vi "Task five.vi"() -> ()   [LabVIEW 2025]
uses:
  <vilib>/httpClient/POSTBuffer.vi
  <vilib>/httpClient/LabVIEWHTTPClient.lvlib
panel:
  in  "User Input":string
  in  "?":bool
  in  "Select correct word":string(combo)
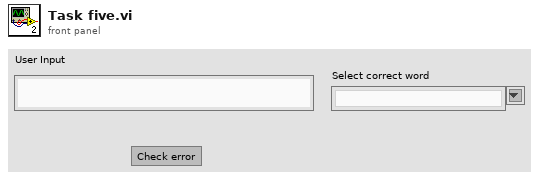
[diagram p1: front panel]
types:
  T1 = cluster{"matches":cluster{"offset":i32, "length":i32, "message":string, "replacements":cluster{"value":string}[]}[]}
  T2 = typedef "LabVIEWHTTPClient.lvlib/ClientHandle.ctl" = refnum<k1>
  T3 = cluster{"offset":i32, "length":i32, "message":string, "replacements":cluster{"value":string}[]}[]
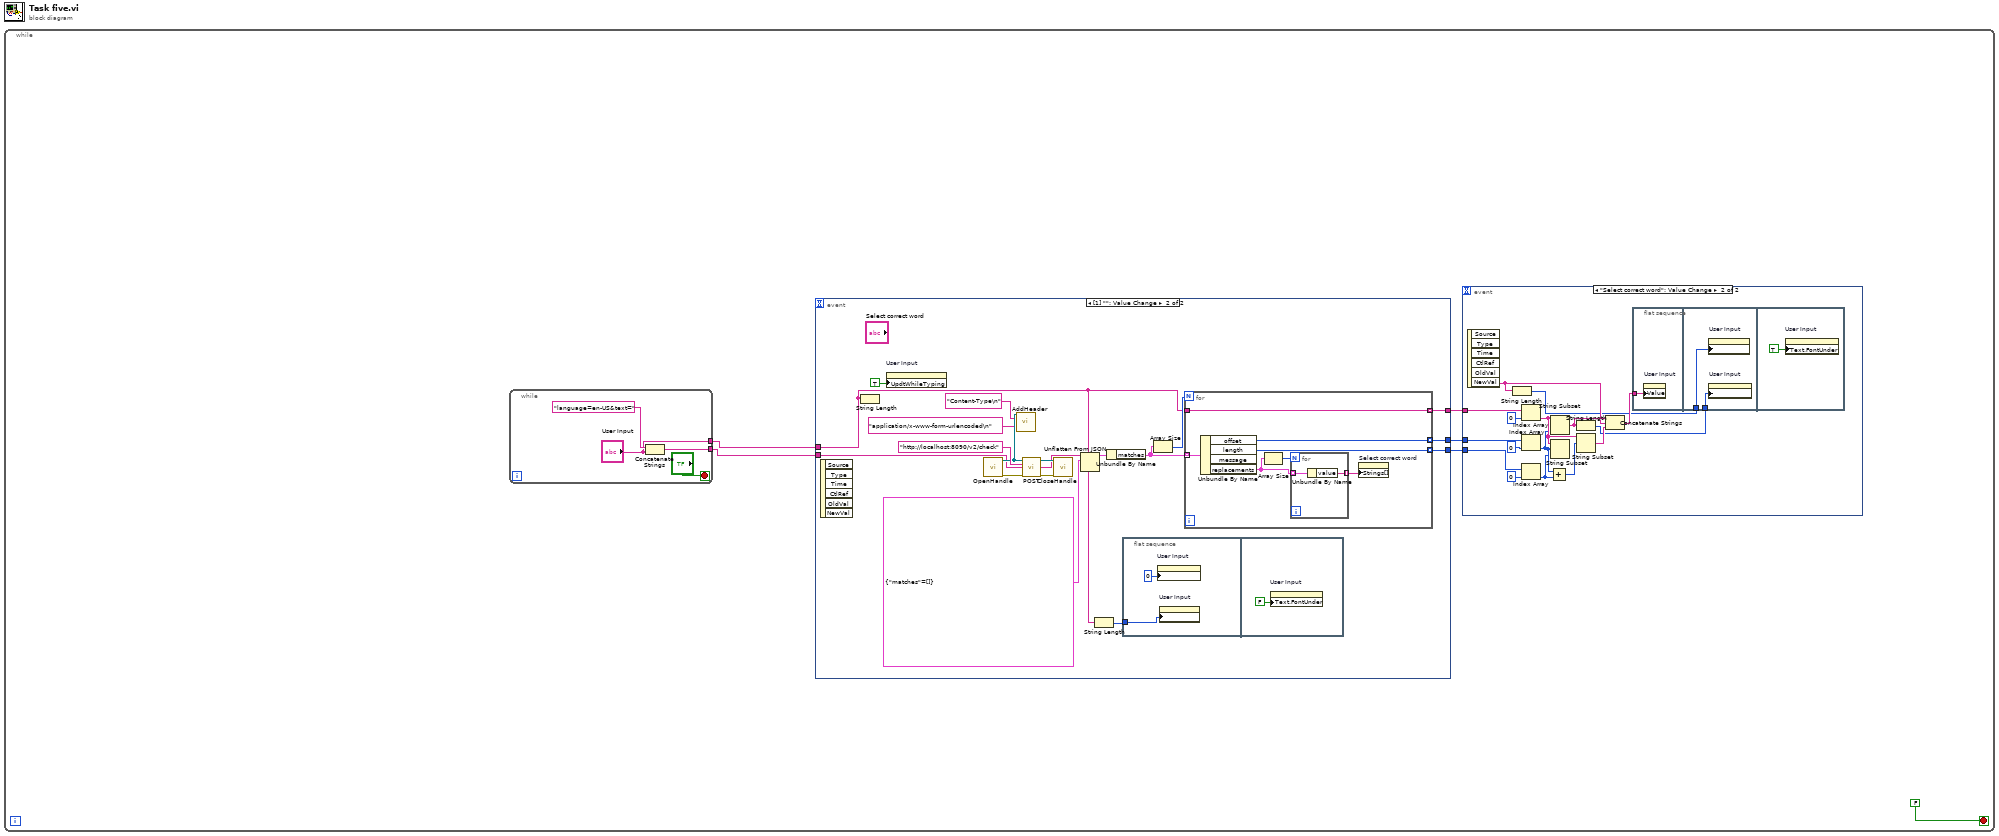
[diagram p0: block diagram]
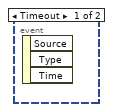
[diagram p2: hidden frame]
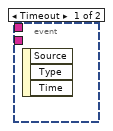
[diagram p3: hidden frame]
diagram:
  n1 = while {
    stop <- FALSE stop-if-true
    n2 = while {
      tunnel: [w9] -> w2
      tunnel: ["User Input"] -> w1
      stop <- "?" stop-if-true
      n3 = Concatenate Strings("language=en-US&text=", "User Input") -> (w9:string)
    }
    n4 = event shown="[1] \"\": Value Change" {
      selector: _ -> [_ _]
      dyn-events: _ -> [_ _]
      timeout: _ -> [_ _]
      tunnel: w2 -> [_ w42]
      tunnel: w1 -> [_ w32]
      tunnel: [_ w36] -> w6
      tunnel: [_ w35] -> w4
      tunnel: [_ w34] -> w5
      event Timeout {
        n5 = event-data() -> ()  [unwired: 1 in, 3 out]
      }
      event Value Change {
        n6 = event-data() -> ()  [unwired: 1 in, 6 out]
        n7 = String Length(string=w32) -> ()  [unwired: 1 out]
        n8 = property on="User Input" class="Str"("UpdtWhileTyping"=TRUE ("Update While Typing?")) -> ()  [unwired: 2 in, 2 out]
        n9 = call <vilib>:"OpenHandle.vi"() -> ("client handle out"=w45:T2, "error out"=w46:errorcluster)  [unwired: 14 in]
        n10 = call <vilib>:"AddHeader.vi"("client handle"=w45, "header"="Content-Type\n", "value"="application/x-www-form-urlencoded\n") -> ()  [unwired: 11 in, 2 out]
        n11 = call-poly <vilib>:"POST.vi"("client handle"=w45, "url"="http://localhost:8090/v2/check", "buffer"=w42, "error in (no error)"=w46) -> ("client handle out"=w48:T2, "body"=w41:string, "error out"=w47:errorcluster)  [unwired: 8 in, 1 out]
        n12 = call <vilib>:"CloseHandle.vi"("client handle"=w48, "error in (no error)"=w47) -> ()  [unwired: 13 in, 1 out]
        n13 = Unflatten From JSON(JSON string=w41, type and defaults=T1 {"matches"=[]}) -> (value=w39:T1)  [unwired: 5 in, 1 out]
        n14 = String Length(string=w32) -> (length=w31:i32)
        n15 = Unbundle By Name(w39) -> ("matches"=w37:T3)
        n16 = flat-sequence {
          tunnel: w31 -> [w50]
          frame #0 {
            n17 = property on="User Input" class="Str"("Text.Selection Start"=u32 0 ("Text.Selection:Start")) -> ()  [unwired: 2 in, 2 out]
            n18 = property on="User Input" class="Str"("Text.Selection End"=w50) -> ()  [unwired: 2 in, 2 out]
          }
          frame #1 {
            n19 = property on="User Input" class="Str"("Text.FontUnder"=FALSE ("Text.Font:Underline")) -> ()  [unwired: 2 in, 2 out]
          }
        }
        n20 = Array Size(array=w37) -> (size(s)=w38:i32)
        n21 = for {
          N: w38 -> [_]
          tunnel: w37 -> [w59] mode=indexing
          tunnel: w32 -> [w53]
          tunnel: [w55] -> w36 mode=indexing
          tunnel: [w53] -> w35 mode=indexing
          tunnel: [w54] -> w34 mode=indexing
          n22 = Unbundle By Name(w59) -> ("offset"=w55:i32, "length"=w54:i32, "replacements"=w57:cluster{"value":string}[])  [unwired: 1 out]
          n23 = Array Size(array=w57) -> (size(s)=w58:i32)
          n24 = for {
            N: w58 -> [_]
            tunnel: w57 -> [w61] mode=indexing
            tunnel: [w60] -> w56 mode=indexing
            n25 = Unbundle By Name(w61) -> ("value"=w60:string)
          }
          n26 = property on="Select correct word" class="CmbBox"("Strings[]"=w56) -> ()  [unwired: 2 in, 2 out]
        }
      }
    }
    n27 = event shown="[1] \"Select correct word\": Value Change" {
      selector: _ -> [_ _]
      dyn-events: _ -> [_ _]
      timeout: _ -> [_ _]
      tunnel: w6 -> [_ w26]
      tunnel: w4 -> [_ w23]
      tunnel: w5 -> [_ w20]
      event Timeout {
        n28 = event-data() -> ()  [unwired: 1 in, 3 out]
      }
      event "Select correct word": Value Change {
        n29 = event-data() -> ("NewVal"=w12:string)  [unwired: 1 in, 5 out]
        n30 = String Length(string=w12) -> (length=w11:i32)
        n31 = Index Array(array=w23, index=0) -> (element=w22:string)
        n32 = Index Array(array=w26, index=0) -> (element=w19:i32)
        n33 = Index Array(array=w20, index=0) -> (element=w18:i32)
        n34 = Add(x=w19, y=w18) -> (x+y=w17:i32)
        n35 = String Subset(string=w22, length (rest)=w19) -> (substring=w14:string)  [unwired: 1 in]
        n36 = String Subset(string=w22, offset (0)=w19, length (rest)=w18) -> ()  [unwired: 1 out]
        n37 = String Length(string=w14) -> (length=w13:i32)
        n38 = String Subset(string=w22, offset (0)=w17) -> (substring=w16:string)  [unwired: 1 in]
        n39 = Concatenate Strings(w14, w12, w16) -> (w15:string)
        n40 = flat-sequence {
          tunnel: w15 -> [w27]
          tunnel: w13 -> [w29]
          tunnel: w11 -> [w28]
          frame #0 {
            n41 = property on="User Input" class="Str"("Value"=w27) -> ()  [unwired: 2 in, 2 out]
          }
          frame #1 {
            n42 = property on="User Input" class="Str"("Text.Selection End"=w28) -> ()  [unwired: 2 in, 2 out]
            n43 = property on="User Input" class="Str"("Text.Selection Start"=w29) -> ()  [unwired: 2 in, 2 out]
          }
          frame #2 {
            n44 = property on="User Input" class="Str"("Text.FontUnder"=TRUE) -> ()  [unwired: 2 in, 2 out]
          }
        }
      }
    }
  }
